vi "nanocal-frontend-tcplink-server -- V2.vi"() -> ()   [LabVIEW 2020]
doc: "Demonstrates how to set up a basic TCP connection, send data to the specified port once a connection has been established, and terminate the connection once the data has been sent. This VI is designed to stop if the TCP connection is terminated. The data sent in this example is an array of random numbers."
uses:
  icicle.ctl
  TCP Multiple Connections example/controls/TCP Multiple Connections State.ctl
  TCP Multiple Connections example/controls/TCP Multiple Connections Data.ctl
  publisher action.ctl
panel:
  out "# of Connections":i32
  in  "Tab Control":enum32{"Page 1", "Page 2"}(tab)
  in  "Stop":bool
  in  "port":u16=6340
  in  "timeout (ms)":i32=30000
  out "nanocal data array OUT":T1[](array[typedef])
  # "nanocal tcplink -- Server"
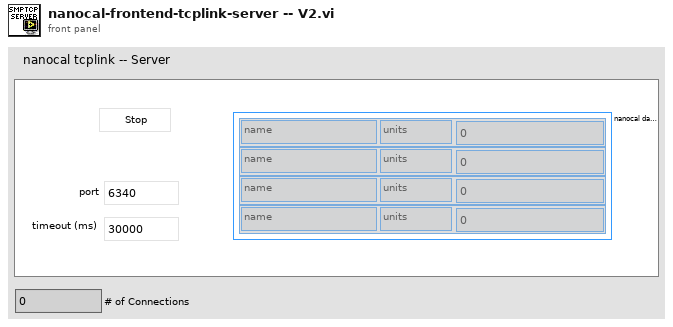
[diagram p1: front panel]
types:
  T1 = typedef "icicle.ctl" = cluster{"name":string, "units":string, "data":dbl}
  T2 = typedef "TCP Multiple Connections Data.ctl" = cluster{"Clients":refnum<k5>[], "Listener":refnum<k5>}
  T3 = typedef "TCP Multiple Connections State.ctl" = enum16{"Initialize", "Status Check", "Send Data", "Stop"}
  T4 = typedef "publisher action.ctl" = enum16{"set", "get", "init", "check"}
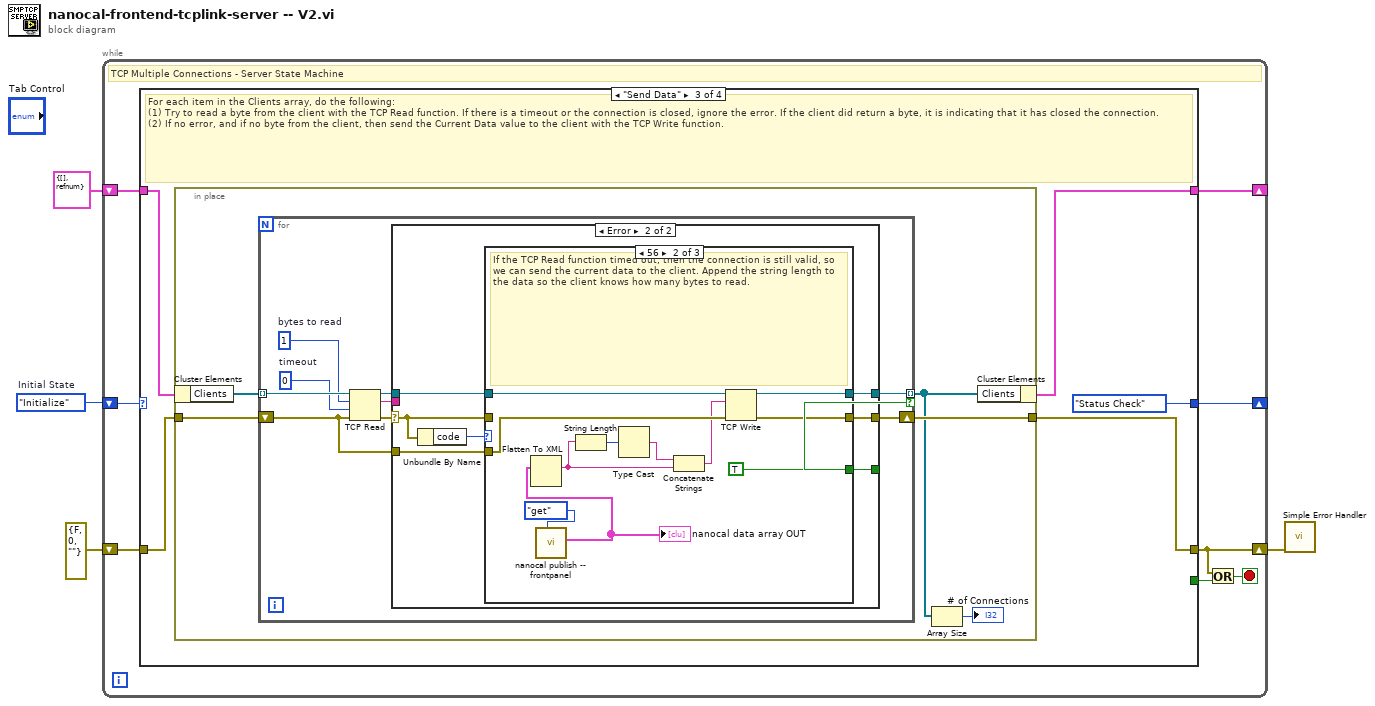
[diagram p0: block diagram]
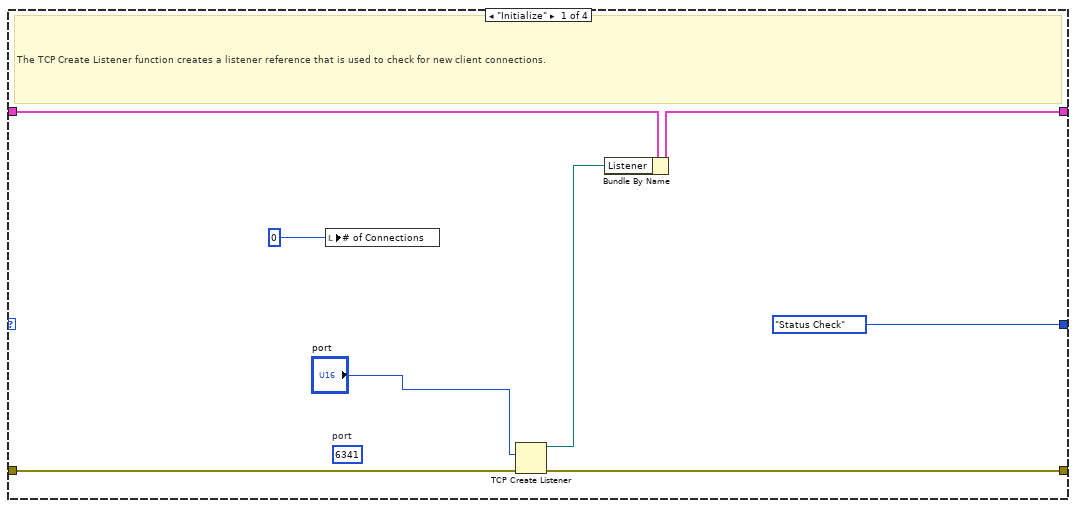
[diagram p2: hidden frame]
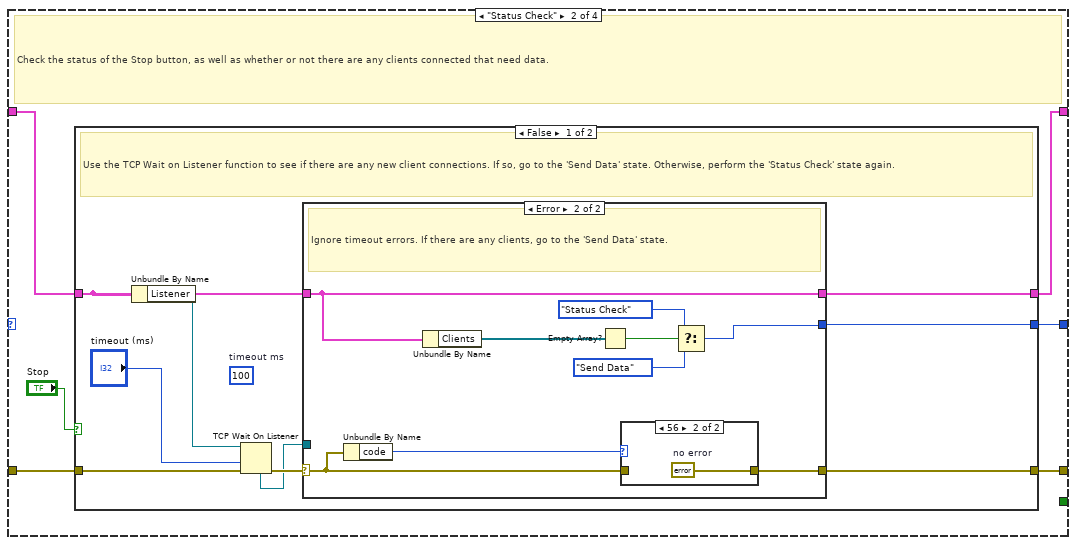
[diagram p3: hidden frame]
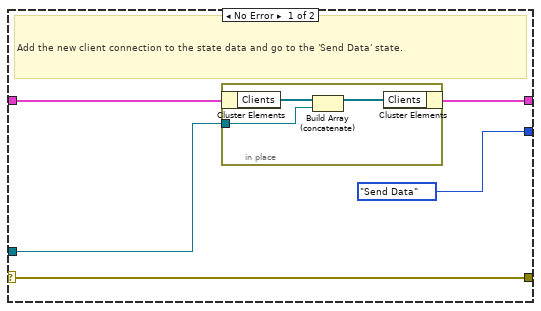
[diagram p4: hidden frame]
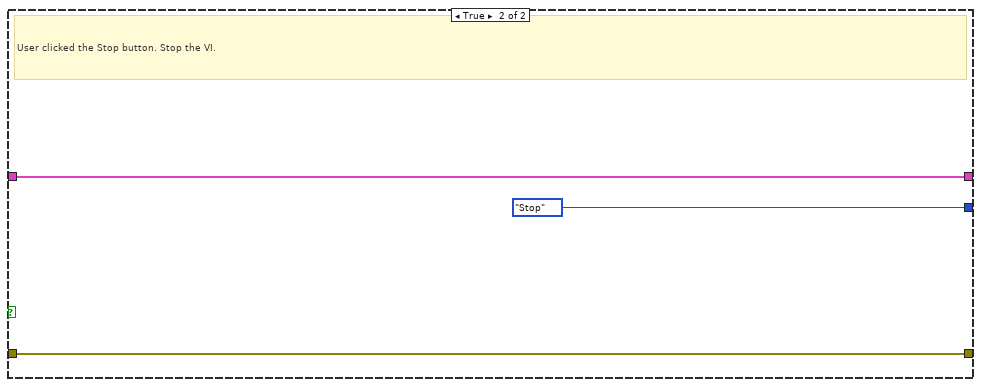
[diagram p6: hidden frame]
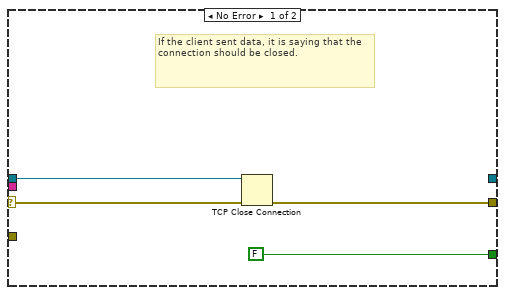
[diagram p7: hidden frame]
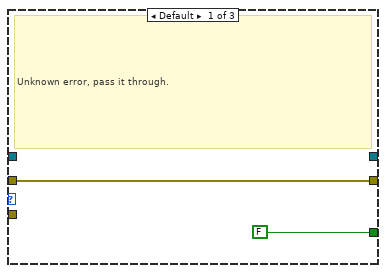
[diagram p8: hidden frame]
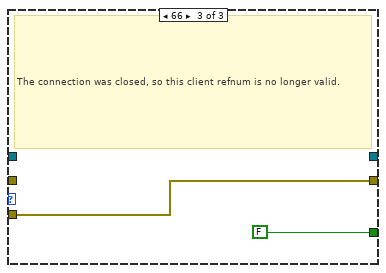
[diagram p9: hidden frame]
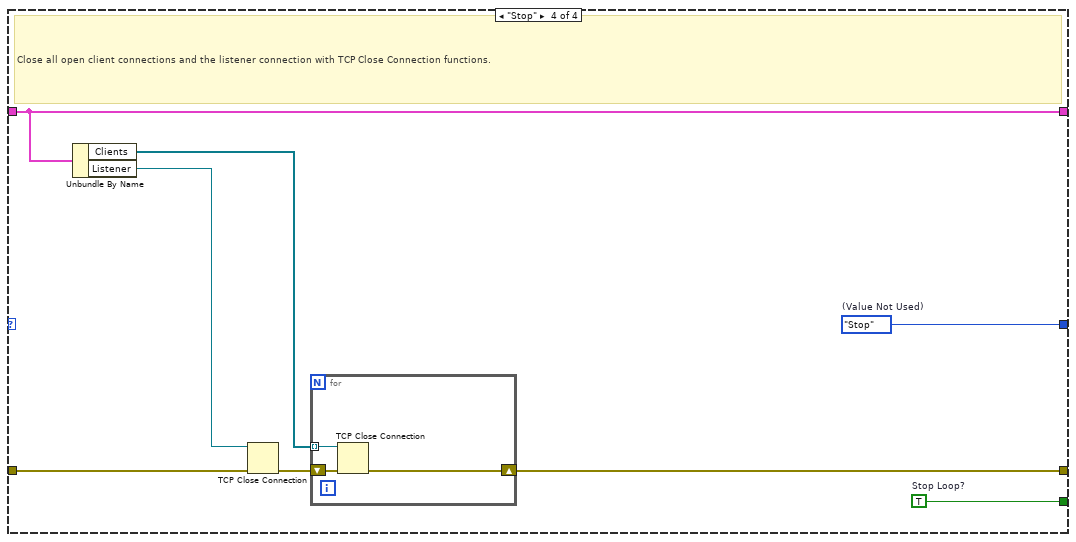
[diagram p10: hidden frame]
diagram:
  w4 = TCP_Multiple_Connections_State."Initialize"  # Initial State
  n1 = while {
    shift-right: [w11] -> _
    shift-left: w4 -> [w12]
    shift-right: [w9] -> _
    shift-left: T2 {"Clients"=[], "Listener"=refnum} ("Data") -> [w10]
    shift-right: [w5] -> w1
    shift-left: errorcluster {"status"=FALSE, "code"=0, "source"=""} ("error constant") -> [w8]
    stop <- w6 stop-if-true
    # "TCP Multiple Connections - Server State Machine"
    n2 = case shown="\"Send Data\"" w12 {
      tunnel: [TCP_Multiple_Connections_State."Status Check" ("States") w26 TCP_Multiple_Connections_State."Status Check" ("States") w104] -> w11
      tunnel: [_ _ _ w111] -> w7
      tunnel: w10 -> [w18 w23 w60 w110]
      tunnel: [w17 w22 w59 w110] -> w9
      tunnel: w8 -> [w20 w25 w62 w109]
      tunnel: [w19 w24 w61 w107] -> w5
      frame "Initialize" {
        (unwired) u16 6341  # port
        # "The TCP Create Listener function creates a listener reference that is used to check for new client connections."
        n3 = local write "# of Connections"(0 ("Number of Client Connections")) -> ()
        n4 = TCP Create Listener(8:w20, 10:"port") -> (0:w19:errorcluster, 3:w16:refnum<k5>)  [unwired: 4 out]
        n5 = Bundle By Name(cluster=w18, "Listener"=w16) -> (w17:T2)
      }
      frame "Status Check" {
        # "Check the status of the Stop button, as well as whether or not there are any clients connected that need data."
        n6 = case shown="False" "Stop" {
          tunnel: [w35 TCP_Multiple_Connections_State."Stop" ("States")] -> w26
          tunnel: w25 -> [w34 w57]
          tunnel: [w28 w57] -> w24
          tunnel: w23 -> [w31 w56]
          tunnel: [w30 w56] -> w22
          frame False {
            (unwired) 100  # timeout ms
            # "Use the TCP Wait on Listener function to see if there are any new client connections. If so, go to the 'Send Data' state. Otherwise, perform the 'Status Check' state again."
            n7 = Unbundle By Name(w31) -> ("Listener"=w29:refnum<k5>)
            n8 = TCP Wait On Listener(8:w34, 9:"timeout (ms)", 11:w29) -> (0:w33:errorcluster, 4:w32:refnum<k5>)  [unwired: 4 out]
            n9 = case shown="Error" w33 {
              selector: w33 -> [w38 w52]
              tunnel: [TCP_Multiple_Connections_State."Send Data" ("States") w46] -> w35
              tunnel: w32 -> [w39 _]
              tunnel: w31 -> [w40 w49]
              tunnel: [w37 w49] -> w30
              tunnel: [w38 w50] -> w28
              frame No Error {
                # "Add the new client connection to the state data and go to the 'Send Data' state."
                n10 = in-place {
                  in-place-border: w39 -> [w41]
                  n11 = in-place-cluster #1(w40) -> ("Clients"=w43:refnum<k5>[])
                  n12 = Build Array (concatenate)(w43, w41) -> (w42:refnum<k5>[])
                  n13 = in-place-cluster #1("Clients"=w42) -> (w37:T2)
                }
              }
              frame Error {
                # "Ignore timeout errors. If there are any clients, go to the 'Send Data' state."
                n14 = Unbundle By Name(w52) -> ("code"=w51:i32)
                n15 = Unbundle By Name(w49) -> ("Clients"=w48:refnum<k5>[])
                n16 = Empty Array?(array=w48) -> (empty?=w47:bool)
                n17 = case shown="56" w51 {
                  tunnel: w52 -> [w53 _]
                  tunnel: [w53 w54] -> w50
                  frame Default {
                  }
                  frame 56 {
                    w54 = errorcluster {"status"=FALSE, "code"=0, "source"=""}  # no error
                  }
                }
                n18 = Select(t=TCP_Multiple_Connections_State."Status Check" ("States"), s=w47, f=TCP_Multiple_Connections_State."Send Data" ("States")) -> (s? t:f=w46:T3)
              }
            }
          }
          frame True {
            # "User clicked the Stop button. Stop the VI."
          }
        }
      }
      frame "Send Data" {
        # "For each item in the Clients array, do the following:\n(1) Try to read a byte from the client with the TCP Read function. If there is a timeout or the connection is closed, ignore the error. If the client did return a byte, it is indicating that it has closed the connection.\n(2) If no error, and if no byte from the client, then send the Current Data value to the client with the TCP Write function."
        n19 = in-place {
          in-place-border: w62 -> [w67]
          in-place-border: [w66] -> w61
          n20 = in-place-cluster #2(w60) -> ("Clients"=w64:refnum<k5>[])
          n21 = for {
            tunnel: w64 -> [w77] mode=indexing
            shift-right: [w69] -> w66
            shift-left: w67 -> [w68]
            tunnel: [w71] -> w63 mode=indexing if=w70
            w74 = 0  # timeout
            w75 = 1  # bytes to read
            n22 = TCP Read(connection ID=w77, bytes to read=w75, error in (no error)=w68, 9:w74) -> (connection ID out=w76:refnum<k5>, data out=w72:string, error out=w73:errorcluster)  [unwired: 1 out]
            n23 = case shown="Error" w73 {
              selector: w73 -> [w80 w87]
              tunnel: w76 -> [w81 w84]
              tunnel: w72 -> [_ _]
              tunnel: [_ w82] -> w71
              tunnel: [FALSE w83] -> w70
              tunnel: [w78 w86] -> w69
              tunnel: w68 -> [_ w85]
              frame No Error {
                # "If the client sent data, it is saying that the connection should be closed."
                # "If the client sent data, it is saying that the connection should be closed."
                n24 = TCP Close Connection(connection ID=w81, error in (no error)=w80) -> (error out=w78:errorcluster)  [unwired: 2 out]
              }
              frame Error {
                # "Ignore connection closed and timeout errors"
                n25 = Unbundle By Name(w87) -> ("code"=w88:i32)
                n26 = case shown="56" w88 {
                  tunnel: w87 -> [w90 _ _]
                  tunnel: [w90 w101 w103] -> w86
                  tunnel: w85 -> [_ w97 w103]
                  tunnel: w84 -> [_ w100 _]
                  tunnel: [FALSE TRUE FALSE] -> w83
                  tunnel: [_ w99 _] -> w82
                  frame Default {
                    # "Unknown error, pass it through."
                  }
                  frame 56 {
                    # "If the TCP Read function timed out, then the connection is still valid, so we can send the current data to the client. Append the string length to the data so the client knows how many bytes to read."
                    n27 = call "nanocal publish -- frontpanel.vi"("publisher action"=publisher_action."get") -> ("nanocal data array OUT"=w95:T1[])  [unwired: 10 in]
                    "nanocal data array OUT" <- w95
                    n28 = Flatten To XML(6:w95) -> (2:w93:string)
                    n29 = String Length(string=w93) -> (length=w96:i32)
                    n30 = Type Cast(x=w96) -> (*(type *) &x=w94:string)  [unwired: 1 out]
                    n31 = Concatenate Strings(w94, w93) -> (w92:string)
                    n32 = TCP Write(connection ID=w100, data in=w92, error in (no error)=w97) -> (connection ID out=w99:refnum<k5>, error out=w101:errorcluster)  [unwired: 2 out]
                  }
                  frame 66 {
                    # "The connection was closed, so this client refnum is no longer valid."
                  }
                }
              }
            }
          }
          n33 = Array Size(array=w63) -> (size(s)=→"# of Connections":i32)
          n34 = in-place-cluster #2("Clients"=w63) -> (w59:T2)
        }
      }
      frame "Stop" {
        w104 = TCP_Multiple_Connections_State."Stop"  # (Value Not Used)
        w111 = TRUE  # Stop Loop?
        # "Close all open client connections and the listener connection with TCP Close Connection functions."
        n35 = Unbundle By Name(w110) -> ("Clients"=w108:refnum<k5>[], "Listener"=w105:refnum<k5>)
        n36 = TCP Close Connection(connection ID=w105, error in (no error)=w109) -> (error out=w106:errorcluster)  [unwired: 1 in, 1 out]
        n37 = for {
          shift-right: [w113] -> w107
          shift-left: w106 -> [w114]
          tunnel: w108 -> [w112] mode=indexing
          n38 = TCP Close Connection(connection ID=w112, error in (no error)=w114) -> (error out=w113:errorcluster)  [unwired: 1 in, 1 out]
        }
      }
    }
    n39 = Or(x=w5, y=w7) -> (x .or. y?=w6:bool)
  }
  n40 = call <vilib>:"Simple Error Handler.vi"("error in (no error)"=w1) -> ()  [unwired: 4 in, 5 out]
